vi "COM Port Initial Dialog.vi"(11 "error in (no error)":errorcluster) -> (8 "OK":bool, 15 "error out":errorcluster)   [LabVIEW 2011]
doc: "Welcome screen, with basic options"
uses:
  Application Structure/Options/Options PageID.ctl
  Application Structure/Options/Action GFV Settings.ctl
panel:
  in  "Modem Status":u16(ring) items=["Select Port", "COM19", "Refresh"]
  in  "Tractor Interface":u16(ring) items=["Select Port", "COM19", "Refresh"]
  in  "Modem Data":u16(ring) items=["Select Port", "COM19", "Refresh"]
  in  "Power Supply/PCP":u16(ring) items=["Select Port", "COM19", "Refresh"]
  in  "Cancel":bool
  in  "OK btn":bool
  # "COM Port Settings Dialog"
  # "Tab header s can be changed as wanted\n\nCustom can be used for completly ccutom behavior,\nmust then highjack  an other hidden page, for settings"
  # "Add custom behavior taht cvan not be replicated by a simple cluster with valisdity checking"
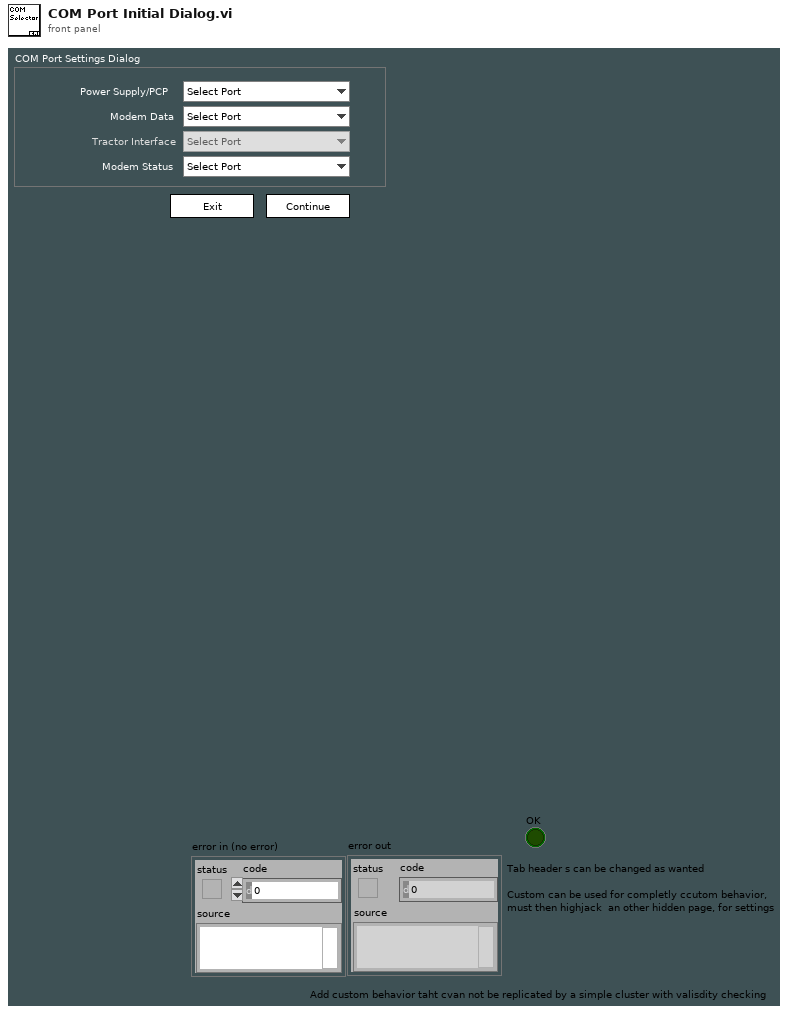
[diagram p1: front panel]
types:
  T1 = enum16{"GET", "SET", "Get from Ini", "Put in Ini"}
  T2 = typedef "Options  All pages and custom.ctl" = cluster{"P 1 (App)":T3, "P 2":T4, "P 3":T5, "P 4":T8, "P 5":T13, "P 6 (Err)":T14, "P 7 (Expert)":T15, "P 8 (Depth)":T17, "C 1":T18, "C 2":T19}
  T3 = typedef "Options Page 1 (App).ctl" = cluster{"Result files":path, "PCP Interface":string, "Tractor/Stroker Interface":string, "Tractor Interface":string, "Modem Status Interface":string, "Audible Alarm":bool, "Force alarm on Technical":bool, "Force alarm on HH":bool, "Force alarm on LL":bool, "Force alarm on H":bool, "Force alarm on L":bool}
  T4 = typedef "Options Page 2.ctl" = cluster{"Solenoid & Relay latching time":u16, "Tractor relay 1":dbl, "Tractor relay 2":dbl, "Tractor Solenoid limit":dbl}
  T5 = typedef "Options Page 3.ctl" = cluster{"Min resistance":dbl, "Max resistance":dbl, "Head voltage range":T6, "Max voltage jump":dbl, "Maximum resistance change":dbl, "Start Telemetry Voltage":dbl, "Start Telemetry Timeout":dbl, "Start Motor Voltage":dbl, "Stop Motor Voltage":dbl, "Pass Mode Warning Voltage":dbl, "Relay Switch Voltage":dbl, "Relay Status Loss Voltage":dbl, "Samples to average":i32, "PSU type DO NOT USE":T7, "Magna OVP":dbl, "Magna Current Limit":dbl}
  T6 = typedef "PCP type List.ctl" = enum16{"0 - 350V", "0 - 450V", "0 - 600V"}
  T7 = typedef "PSU Type.ctl" = enum16{"Unipower", "Magna 8.3A", "Magna 12A", "None"}
  T8 = typedef "Options Page 4.ctl" = cluster{"Solenoid & Relay latching time":u16, "Stroker relay 1":dbl, "Stroker Relay 2":dbl, "Stroker Solenoid limit":dbl, "Force det.":T9, "Stroke force lim.":dbl, "Anchor Enabled Pressure":dbl, "Tacometer puls":dbl, "Default anchor behavior":T10, "Default stroker behavior":T11, "Default stroker force limit (tonne)":dbl, "Slips Size":T12}
  T9 = typedef "Stroke force selector.ctl" = enum16{"Stroke in = node 1", "Strok out = node 1"}
  T10 = typedef "Default anchor behavior.ctl" = enum16{"Do nothing", "Set Anchor", "Release Anchor"}
  T11 = typedef "Default stroker behavior.ctl" = enum16{"Do nothing", "Stop", "Go Out", "Go In"}
  T12 = typedef "Slips Type Radio.ctl" = enum32{"No Selection", "338 MRS", "3,9 MRS"}
  T13 = typedef "Options Page 5.ctl" = cluster{"Solenoid & Relay latching time":u16, "Driller relay 1":dbl, "Driller Relay 2":dbl, "Driller  Solenoid limit":dbl}
  T14 = typedef "Options Page 6 (Err).ctl" = cluster{"Error and event files":path}
  T15 = typedef "Options Page 7 (Expert).ctl" = cluster{"Show Debug":bool, "Log debug messages":bool, "Additional debug messages":bool, "Start Beagle with Simulator data":bool, "Workshop mode":bool, "Modem baud":u16, "enumCANCOM":bool, "Modem sim":T16, "Telemetry Timeout Disable":i32, "Buffer size":i32, "Upd regular data":bool, "Cable comp":cluster{"VMOD1 Voltage(V)":dbl, "VMOD2 Voltage(V)":dbl}}
  T16 = typedef "Modem simulation setup.ctl" = cluster{"Modem dealay sim":bool, "Sim baud Tx":u16, "Bit Error fraction Tx":dbl, "Sim baud Rx":u16, "Bit Error fraction Rx":dbl}
  T17 = typedef "Options Page 8 (Depth).ctl" = cluster{"Winch Spool Circumference":dbl, "Winch Pulses per Revolution":dbl, "Current Depth":dbl}
  T18 = typedef "Options Custom 1.ctl" = cluster{"Depth Updated":bool, "Depth Offset":dbl}
  T19 = typedef "Options Custom 2.ctl" = cluster{"Placeholder":bool}
  T20 = typedef "Options PageID.ctl" = enum16{"P 1 (App)", "P 2", "P 3", "P 4", "P 5", "P 6 (Err)", "P 7 (Expert)", "P 8", "C 1", "C 2"}
  T21 = typedef "Action GFV Settings.ctl" = enum16{"Init", "Get From INI", "Put In INI", "Get Settings", "Get Update Index", "Set Setting"}
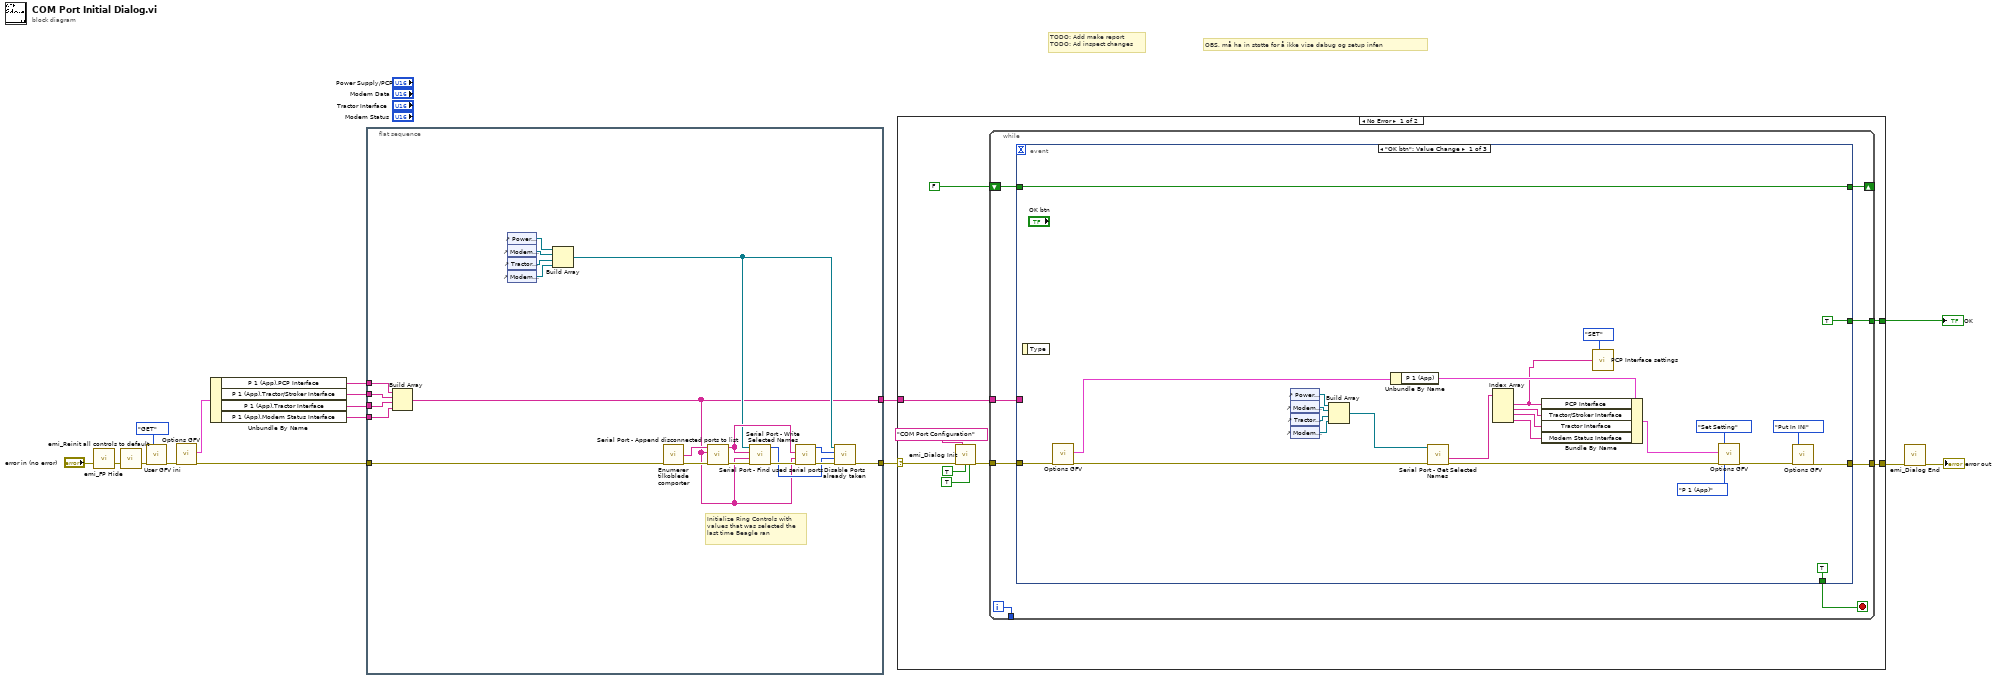
[diagram p0: block diagram]
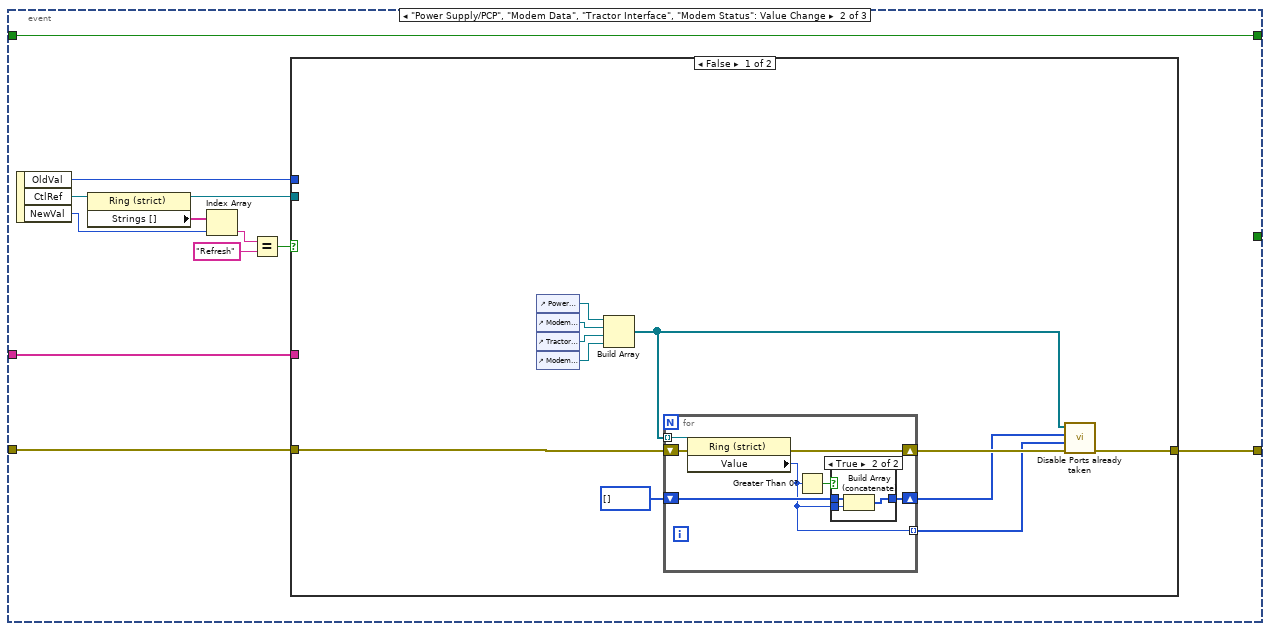
[diagram p2: hidden frame]
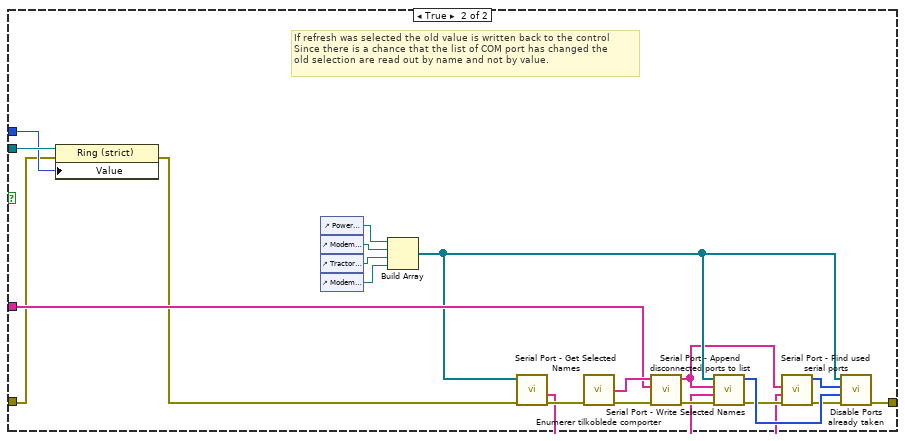
[diagram p4: hidden frame]
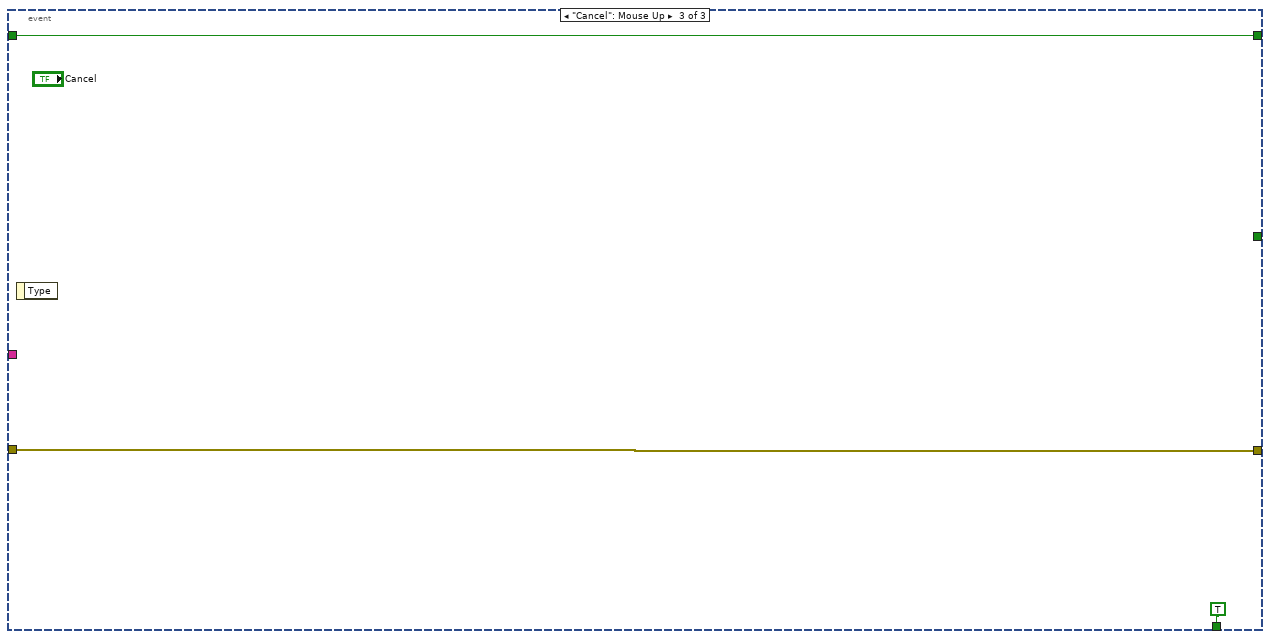
[diagram p5: hidden frame]
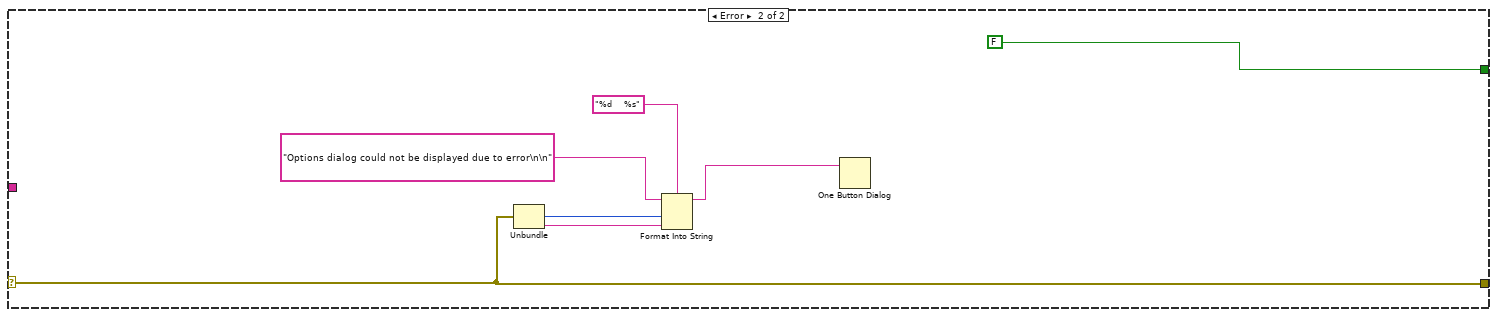
[diagram p6: hidden frame]
diagram:
  # "OBS, må ha in støtte for å ikke vise dabug og setup infen"
  # "TODO: Add make report\nTODO: Ad inspect changes"
  n1 = call "emi_FP Hide.vi"("error in (no error)"="error in (no error)") -> ("error out"=w4:errorcluster)  [unwired: 13 in, 1 out]
  n2 = call "emi_Reinit all controls to default.vi"("error in (no error)"=w4) -> ("error out"=w2:errorcluster)  [unwired: 13 in, 1 out]
  n3 = call "User GFV ini.vi"("Action(GET)"=T1."GET", "error in (no error)"=w2) -> ("error out"=w12:errorcluster)  [unwired: 12 in, 1 out]
  n4 = call "Options GFV.vi"("error in (no error)"=w12) -> ("Options"=w7:T2, "error out"=w11:errorcluster)  [unwired: 16 in, 1 out]
  n5 = Unbundle By Name(w7) -> ("P 1 (App).PCP Interface"=w10:string, "P 1 (App).Tractor/Stroker Interface"=w9:string, "P 1 (App).Tractor Interface"=w8:string, "P 1 (App).Modem Status Interface"=w6:string)
  n6 = flat-sequence {
    tunnel: [w20] -> w13
    tunnel: w11 -> [w18]
    tunnel: w10 -> [w36]
    tunnel: w9 -> [w35]
    tunnel: w8 -> [w34]
    tunnel: w6 -> [w33]
    tunnel: [w17] -> w1
    frame #0 {
      # "Initialize Ring Controls with \nvalues that was selected the\nlast time Beagle ran"
      n7 = Build Array(w36, w35, w34, w33) -> (w17:string[])
      n8 = control-ref of="Power Supply/PCP"() -> (w32:refnum<vi>)
      n9 = control-ref of="Modem Data"() -> (w31:refnum<vi>)
      n10 = control-ref of="Tractor Interface"() -> (w30:refnum<vi>)
      n11 = control-ref of="Modem Status"() -> (w29:refnum<vi>)
      n12 = Build Array(w32, w31, w30, w29) -> (w19:refnum<vi>[])
      n13 = call "Enumerer tilkoblede comporter.vi"("error in (no error)"=w18) -> ("Com port w Select string"=w24:string[], "error out"=w23:errorcluster)  [unwired: 11 in, 2 out]
      n14 = call "Serial Port - Append disconnected ports to list.vi"("error in (no error)"=w23, "Selected Values"=w17, "Connected COM Ports in"=w24) -> ("error out"=w26:errorcluster, "COM Ports out"=w25:string[])  [unwired: 7 in]
      n15 = call "Serial Port - Write Selected Names.vi"("error in (no error)"=w26, "Selected Names"=w17, "COM Port List"=w25, "Ctrl Refs in"=w19) -> ("error out"=w27:errorcluster, "Selected Values"=w21:i32[])  [unwired: 6 in]
      n16 = call "Serial Port - Find used serial ports.vi"("error in (no error)"=w27, "Selected Values"=w17, "COM Ports list"=w25) -> ("error out"=w28:errorcluster, "Items to disable"=w22:i32[])  [unwired: 7 in]
      n17 = call "Disable Ports already taken.vi"("error in (no error)"=w28, "Values"=w21, "COM Port numbers taken"=w22, "Ctrl References"=w19) -> ("error out"=w20:errorcluster)  [unwired: 7 in]
    }
  }
  n18 = case shown="No Error" w13 {
    selector: w13 -> [w40 w142]
    tunnel: [w45 FALSE] -> w16
    tunnel: [w44 w142] -> w15
    tunnel: w1 -> [w37 _]
    frame No Error {
      n19 = call "emi_Dialog Init.vi"("Header String(\"\")"="COM Port Configuration" ("Header String(\"\")"), "error in"=w40, "Set BG Color(T)"=TRUE, "Modal(T)"=TRUE) -> ("error out"=w43:errorcluster)  [unwired: 11 in]
      n20 = while {
        tunnel: [w53] -> _
        tunnel: w43 -> [w51]
        tunnel: [w50] -> w44
        tunnel: [w49] -> w45
        shift-right: [w47] -> _
        shift-left: FALSE -> [w48]
        tunnel: w37 -> [w46]
        i -> [w53]
        stop <- w52 stop-if-true
        n21 = event shown="[0] \"OK btn\": Value Change" {
          selector: _ -> [_ _ _]
          dyn-events: _ -> [_ _ _]
          timeout: _ -> [_ _ _]
          tunnel: [TRUE _ TRUE] -> w52
          tunnel: w51 -> [w75 w89 w135]
          tunnel: [w74 w88 w135] -> w50
          tunnel: [TRUE _ _] -> w49
          tunnel: w48 -> [w77 w90 w134]
          tunnel: [w77 w90 w134] -> w47
          tunnel: w46 -> [_ w79 _]
          event "OK btn": Value Change {
            n22 = event-data() -> ()  [unwired: 1 in, 1 out]
            n23 = call "Options GFV.vi"("error in (no error)"=w75) -> ("Options"=w73:T2, "error out"=w57:errorcluster)  [unwired: 16 in, 1 out]
            n24 = control-ref of="Power Supply/PCP"() -> (w62:refnum<vi>)
            n25 = control-ref of="Modem Data"() -> (w63:refnum<vi>)
            n26 = control-ref of="Tractor Interface"() -> (w64:refnum<vi>)
            n27 = control-ref of="Modem Status"() -> (w65:refnum<vi>)
            n28 = Build Array(w62, w63, w64, w65) -> (w58:refnum<vi>[])
            n29 = Unbundle By Name(w73) -> ("P 1 (App)"=w68:T3)
            n30 = call "Serial Port - Get Selected Names.vi"("error in (no error)"=w57, "Ctrl Refs in"=w58) -> ("error out"=w66:errorcluster, "Selected Names"=w56:string[])  [unwired: 8 in]
            n31 = Index Array(array=w56) -> (element #1=w54:string, element #2=w61:string, element #3=w60:string, element #4=w59:string)  [unwired: 4 in]
            n32 = Bundle By Name(cluster=w68, "PCP Interface"=w54, "Tractor/Stroker Interface"=w61, "Tractor Interface"=w60, "Modem Status Interface"=w59) -> (w67:T3)
            n33 = call "PCP Interface settings.vi"("Action(GET)"=enum16{"GET", "SET"}."SET", "PCP VISA  name  in"=w54) -> ()  [unwired: 12 in, 2 out]
            n34 = call "Options GFV.vi"("Anything"=w67, "error in (no error)"=w66, "Action(Get Settings)"=Action_GFV_Settings."Set Setting", "Setting ID"=Options_PageID."P 1 (App)") -> ("error out"=w72:errorcluster)  [unwired: 13 in, 2 out]
            n35 = call "Options GFV.vi"("error in (no error)"=w72, "Action(Get Settings)"=Action_GFV_Settings."Put In INI") -> ("error out"=w74:errorcluster)  [unwired: 15 in, 2 out]
          }
          event "Power Supply/PCP", "Modem Data", "Tractor Interface", "Modem Status": Value Change {
            n36 = event-data() -> ("OldVal"=w81:u16, "CtlRef"=w87:refnum<vi>, "NewVal"=w85:u16)  [unwired: 1 in]
            n37 = property class="Ring (strict)"(reference=w87) -> (reference out=w80:refnum<vi>, "Strings []"=w86:string[])  [unwired: 1 in, 1 out]
            n38 = Index Array(array=w86, index=w85) -> (element=w84:string)
            n39 = Equal?(x=w84, y="Refresh") -> (x = y?=w82:bool)
            n40 = case shown="False" w82 {
              tunnel: w89 -> [w93 w121]
              tunnel: [w92 w127] -> w88
              tunnel: w81 -> [_ w132]
              tunnel: w80 -> [_ w133]
              tunnel: w79 -> [_ w126]
              frame False {
                n41 = control-ref of="Power Supply/PCP"() -> (w99:refnum<vi>)
                n42 = control-ref of="Modem Data"() -> (w100:refnum<vi>)
                n43 = control-ref of="Tractor Interface"() -> (w101:refnum<vi>)
                n44 = control-ref of="Modem Status"() -> (w91:refnum<vi>)
                n45 = Build Array(w99, w100, w101, w91) -> (w96:refnum<vi>[])
                n46 = for {
                  tunnel: w96 -> [w108] mode=indexing
                  shift-right: [w107] -> w97
                  shift-left: w93 -> [w106]
                  tunnel: [w103] -> w94 mode=indexing
                  shift-right: [w105] -> w95
                  shift-left: i32[] [] -> [w104]
                  n47 = property class="Ring (strict)"(reference=w108, error in=w106) -> (error out=w107:errorcluster, "Value"=w103:u16)  [unwired: 1 out]
                  n48 = Greater Than 0?(x=w103) -> (x > 0?=w102:bool)
                  n49 = case shown="True" w102 {
                    tunnel: w103 -> [_ w112]
                    tunnel: [w109 w111] -> w105
                    tunnel: w104 -> [w109 w110]
                    frame False {
                    }
                    frame True {
                      n50 = Build Array (concatenate)(w110, w112) -> (w111:i32[])
                    }
                  }
                }
                n51 = call "Disable Ports already taken.vi"("error in (no error)"=w97, "Values"=w94, "COM Port numbers taken"=w95, "Ctrl References"=w96) -> ("error out"=w92:errorcluster)  [unwired: 7 in]
              }
              frame True {
                # "If refresh was selected the old value is written back to the control\nSince there is a chance that the list of COM port has changed the \nold selection are read out by name and not by value."
                n52 = property class="Ring (strict)"(reference=w133, error in=w121, "Value"=w132) -> (error out=w120:errorcluster)  [unwired: 1 out]
                n53 = control-ref of="Power Supply/PCP"() -> (w122:refnum<vi>)
                n54 = control-ref of="Modem Data"() -> (w123:refnum<vi>)
                n55 = control-ref of="Tractor Interface"() -> (w124:refnum<vi>)
                n56 = control-ref of="Modem Status"() -> (w125:refnum<vi>)
                n57 = Build Array(w122, w123, w124, w125) -> (w118:refnum<vi>[])
                n58 = call "Serial Port - Get Selected Names.vi"("error in (no error)"=w120, "Ctrl Refs in"=w118) -> ("error out"=w119:errorcluster, "Selected Names"=w113:string[])  [unwired: 8 in]
                n59 = call "Enumerer tilkoblede comporter.vi"("error in (no error)"=w119) -> ("Com port w Select string"=w128:string[], "error out"=w129:errorcluster)  [unwired: 11 in, 2 out]
                n60 = call "Serial Port - Append disconnected ports to list.vi"("error in (no error)"=w129, "Selected Values"=w126, "Connected COM Ports in"=w128) -> ("error out"=w116:errorcluster, "COM Ports out"=w117:string[])  [unwired: 7 in]
                n61 = call "Serial Port - Write Selected Names.vi"("error in (no error)"=w116, "Selected Names"=w113, "COM Port List"=w117, "Ctrl Refs in"=w118) -> ("error out"=w115:errorcluster, "Selected Values"=w131:i32[])  [unwired: 6 in]
                n62 = call "Serial Port - Find used serial ports.vi"("error in (no error)"=w115, "Selected Values"=w113, "COM Ports list"=w117) -> ("error out"=w114:errorcluster, "Items to disable"=w130:i32[])  [unwired: 7 in]
                n63 = call "Disable Ports already taken.vi"("error in (no error)"=w114, "Values"=w131, "COM Port numbers taken"=w130, "Ctrl References"=w118) -> ("error out"=w127:errorcluster)  [unwired: 7 in]
              }
            }
          }
          event "Cancel": Mouse Up {
            n64 = event-data() -> ()  [unwired: 1 in, 1 out]
          }
        }
      }
    }
    frame Error {
      n65 = Unbundle(w142) -> ("code"=w139:i32, "source"=w138:string)  [unwired: 1 out]
      n66 = Format Into String(format string="%d    %s", initial string="Options dialog could not be displayed due to error\n\n" ("message"), w139, w138) -> (resulting string=w140:string)  [unwired: 1 in, 1 out]
      n67 = One Button Dialog(message=w140) -> ()  [unwired: 1 in, 1 out]
    }
  }
  "OK" <- w16
  n68 = call "emi_Dialog End.vi"("error in"=w15) -> ("error out"=→"error out":errorcluster)  [unwired: 14 in]
